vi "Configure Replay Screen.vi"(8 "error in (no error)":errorcluster, 10 "Screen Index (0)":i32, 11 "VISA resource name":refnum<visa-resource-name>) -> (0 "error out":errorcluster, 3 "VISA resource name out":refnum<visa-resource-name>)   [LabVIEW 2014, in "Fluke 190 Series II.lvlib"]
doc: "Selects and setups the Replay analysis mode, and selects and brings on to the instrument's screen a user-selected replay screen-image from memory."
uses:
  Fluke 190 Series II.lvlib
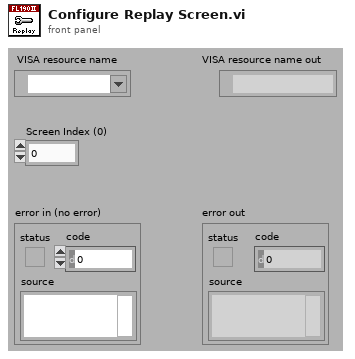
[diagram p1: front panel]
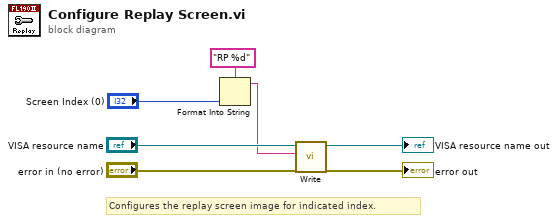
[diagram p0: block diagram]
diagram:
  # "Configures the replay screen image for indicated index."
  n1 = Format Into String(format string="RP %d", "Screen Index (0)") -> (resulting string=w1:string)  [unwired: 2 in, 1 out]
  n2 = call "Write.vi"("error in (no error)"="error in (no error)", "Write Buffer"=w1, "VISA resource name"="VISA resource name") -> ("error out"=→"error out":errorcluster, "VISA resource name out"=→"VISA resource name out":refnum<visa-resource-name>)  [unwired: 7 out]
